vi "Write Title Bar.vi"(10 "Title Bar":bool, 11 "Flex Dialog in":refnum<class "Flex UI Dialog.lvclass">) -> (3 "Flex Dialog out":refnum<class "Flex UI Dialog.lvclass">)   [LabVIEW 2016, in "Flex UI Dialog.lvclass"]
uses:
  Flex UI Dialog.lvclass
  Flex UI Dialog.lvclass/Flex UI Dialog.ctl
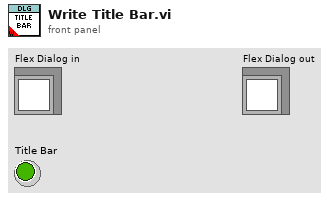
[diagram p1: front panel]
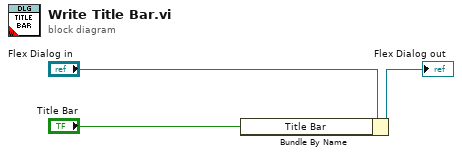
[diagram p0: block diagram]
diagram:
  n1 = Bundle By Name(cluster="Flex Dialog in", "Title Bar"="Title Bar") -> (→"Flex Dialog out":refnum<class "Flex UI Dialog.lvclass">)
